vi "Sensor Data Compiled Multiple Servers.vi"() -> ()   [LabVIEW 2019]
uses:
  <vilib>/Utility/file.llb/Write Delimited Spreadsheet (string).vi
panel:
  in  "URLs":string[](array[string])
  out "data":string
  in  "error in":errorcluster
  out "error out":errorcluster
  out "data cut":string
  out "Labels":string[](array[string])
  out "Values (STR)":string[](array[string])
  in  "stop":bool
  in  "file path (dialog if empty)":path
  out "Table":string[][](table)
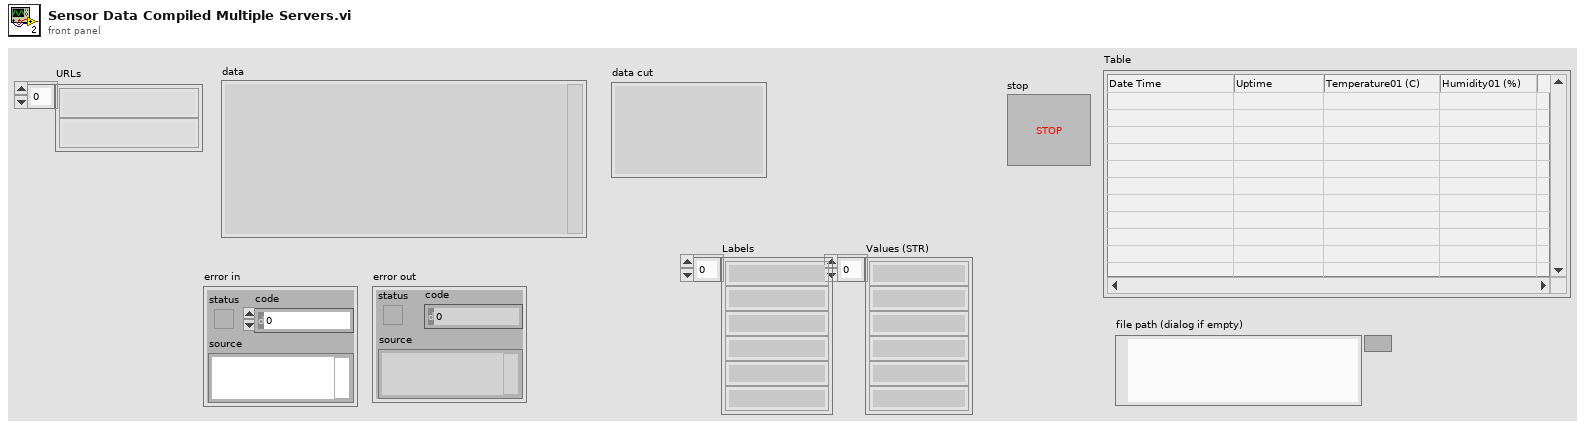
[diagram p1: front panel]
types:
  T1 = enum16{"Read", "Write", "ReadWrite", "BufferedRead", "BufferedReadWrite"}
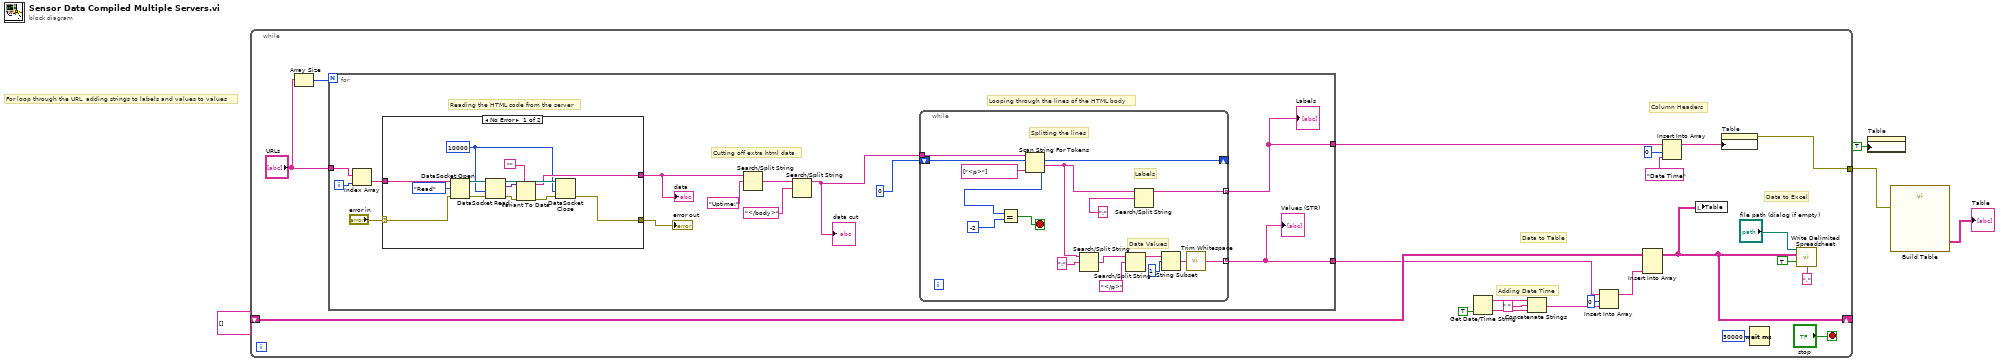
[diagram p0: block diagram]
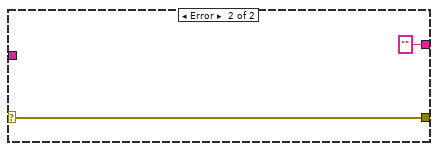
[diagram p2: hidden frame]
diagram:
  # "For loop through the URL, adding strings to labels and values to values"
  n1 = while {
    tunnel: [w26] -> w4
    shift-right: [w10] -> _
    shift-left: string[][] [] -> [w21]
    stop <- "stop" stop-if-true
    # "Data to Excel"
    # "Adding Date Time"
    # "Data to Table"
    # "Column Headers"
    n2 = Array Size(array="URLs") -> (size(s)=w7:i32)
    n3 = for {
      N: w7 -> [_]
      tunnel: [w31] -> w5
      tunnel: [w30] -> w18
      tunnel: "URLs" -> [w27]
      i -> [w28]
      # "Looping through the lines of the HTML body"
      # "Cutting off extra html data"
      # "Reading the HTML code from the server"
      n4 = Index Array(array=w27, index=w28) -> (element=w29:string)
      n5 = case shown="No Error" "error in" {
        selector: "error in" -> [w58 w71]
        tunnel: w29 -> [w62 _]
        tunnel: [w60 ""] -> w37
        tunnel: [w57 w71] -> w39
        frame No Error {
          w59 = 10000 ("ms timeout (10000)")
          n6 = DataSocket Open(8:w58, 10:T1."Read" ("mode"), 11:w62) -> (0:w66:errorcluster, 3:w69:refnum<k13>)  [unwired: 1 out]
          n7 = DataSocket Read(8:w66, 9:w59, 11:w69) -> (0:w67:errorcluster, 2:w64:variant, 3:w68:refnum<k13>)  [unwired: 2 in, 4 out]
          n8 = Variant To Data(error in=w67, type="", Variant=w64) -> (data=w60:string, error out=w65:errorcluster)
          n9 = DataSocket Close(8:w65, 9:w59, 11:w68) -> (0:w57:errorcluster)  [unwired: 1 out]
        }
        frame Error {
        }
      }
      "data" <- w37
      "error out" <- w39
      n10 = Search/Split String(string=w37, search string/char (-)="Uptime:") -> (match + rest of string=w35:string)  [unwired: 1 in, 2 out]
      n11 = Search/Split String(string=w35, search string/char (-)="</body>") -> (substring before match=w32:string)  [unwired: 1 in, 2 out]
      "data cut" <- w32
      n12 = while {
        shift-right: [w54] -> _
        shift-left: 0 -> [w55]
        tunnel: w32 -> [w56]
        tunnel: [w48] -> w31 mode=indexing
        tunnel: [w43] -> w30 mode=indexing
        stop <- w51 stop-if-true
        # "Data Values"
        # "Labels"
        # "Splitting the lines"
        n13 = Scan String For Tokens(6:string[] ["<p>"] ("delimiters (\\s,\\t,\\r,\\n)"), 8:w55, 9:w56) -> (0:w52:i32, 1:w46:string, 2:w54:i32)  [unwired: 3 in, 1 out]
        n14 = Equal?(x=w52, y=-2) -> (x = y?=w51:bool)
        n15 = Search/Split String(string=w46, search string/char (-)=":") -> (match + rest of string=w44:string)  [unwired: 1 in, 2 out]
        n16 = Search/Split String(string=w44, search string/char (-)="</p>") -> (substring before match=w41:string)  [unwired: 1 in, 2 out]
        n17 = Search/Split String(string=w46, search string/char (-)=":") -> (substring before match=w48:string)  [unwired: 1 in, 2 out]
        n18 = String Subset(string=w41, offset (0)=1) -> (substring=w42:string)  [unwired: 1 in]
        n19 = call <vilib>:"Trim Whitespace.vi"("string"=w42) -> ("trimmed string"=w43:string)  [unwired: 1 in]
      }
      "Values (STR)" <- w30
      "Labels" <- w31
    }
    n20 = Get Date/Time String(want seconds? (F)=TRUE) -> (date string=w13:string, time string=w16:string)  [unwired: 2 in]
    n21 = Concatenate Strings(w13, " " ("string"), w16) -> (w14:string)
    n22 = Insert Into Array(array=w18, index=0, new element=w14) -> (w17:string[])
    n23 = Insert Into Array(array=w21, new element=w17) -> (w10:string[][])  [unwired: 2 in]
    n24 = Insert Into Array(array=w5, index=0, new element="Date Time" ("new element/subarray")) -> (w23:string[])
    n25 = local write "Table"(w10) -> ()
    n26 = property on="Table" class="Tbl (strict)"("Column Headers[]"=w23) -> (error out=w26:errorcluster)  [unwired: 2 in, 1 out]
    n27 = Wait (ms)(milliseconds to wait=u32 30000) -> ()  [unwired: 1 out]
    n28 = call-poly <vilib>:"Write Delimited Spreadsheet.vi"("file path (dialog if empty)"="file path (dialog if empty)", "2D data"=w10, "append to file? (new file:F)"=TRUE, "delimiter (\\t)"="," ("delimiter (\\t)")) -> ()  [unwired: 10 in, 2 out]
  }
  n29 = property on="Table" class="Tbl (strict)"("Col Headers Vis"=TRUE ("Visible Items:Column Headers Visible")) -> ()  [unwired: 2 in, 2 out]
  n30 = call "Build Table"("error in (no error)"=w4) -> ("Table"=→"Table":string[][])  [unwired: 4 in, 6 out]
